vi "Pockels Cal-Wizard.vi"   [LabVIEW 2013]
uses:
  Configuration code/Calibration/AOL Z/Typedefs/Cal points.ctl
  User Interface/Windows/System config window/Typedefs/HW Setup tab control.ctl
  Configuration code/Calibration/Globals/gl_Calibration globals.vi
types:
  T1 = enum8{"Enabled", "Disabled", "Disabled and Grayed Out"}
  T2 = typedef "HW Setup tab control.ctl" = enum32{"Control system ", "Triggers", "DAQ FPGA", "HW Channels Setup", "XY stage", "Encoder", "System Setup", "Cameras", "AOL Properties", "Calibration Settings", "Reserved 1", "Reserved 2"}
  T3 = typedef "Cal points.ctl" = enum16{"5-points calibration (crude)", "11-points calibration", "21-points calibration", "41-points calibration"}
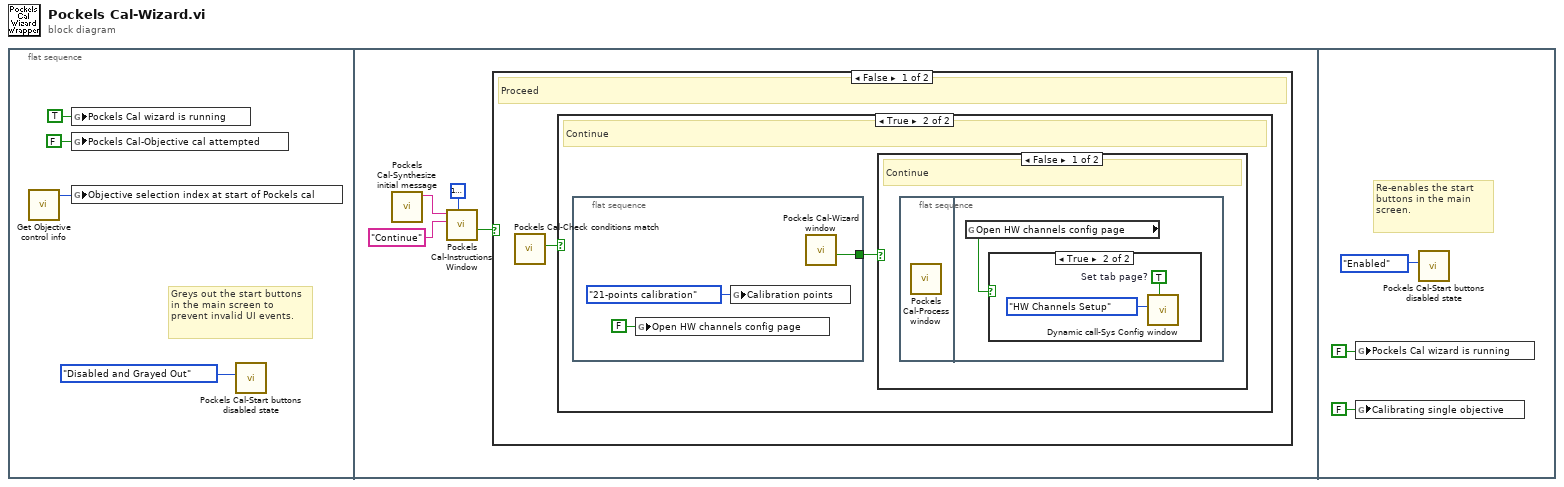
[diagram p0: block diagram]
diagram:
  n1 = flat-sequence {
    frame #0 {
      # "Greys out the start buttons in the main screen to prevent invalid UI events."
      n2 = call "Get Objective control info.vi"() -> ("Selection index"=w1:i32)  [unwired: 7 in, 4 out]
      n3 = global write "gl_Calibration globals.vi" "Pockels Cal wizard is running"(TRUE ("Motor Z Cal wizard is running")) -> ()
      n4 = global write "gl_Calibration globals.vi" "Pockels Cal-Objective cal attempted"(FALSE ("Pockels Cal-Objective cal attempted")) -> ()
      n5 = global write "gl_Calibration globals.vi" "Objective selection index at start of Pockels cal"(w1) -> ()
      n6 = call "Pockels Cal-Start buttons disabled state.vi"("Disabled"=T1."Disabled and Grayed Out") -> ()  [unwired: 10 in, 1 out]
    }
    frame #1 {
      n7 = call "Pockels Cal-Synthesize initial message.vi"() -> ("Message"=w6:string)  [unwired: 11 in]
      n8 = call "Pockels Cal-Instructions Window.vi"("Colour"=u32 16777225, "Caption-Right button (OK)"="Continue", "Message string"=w6) -> ("Cancelled (Left button pressed)"=w8:bool)  [unwired: 7 in, 1 out]
      n9 = case shown="False" w8 {
        frame False {
          # "Proceed"
          n10 = call "Pockels Cal-Check conditions match.vi"() -> ("Continue"=w9:bool)  [unwired: 11 in]
          n11 = case shown="True" w9 {
            frame False {
              # "Cancelled"
            }
            frame True {
              # "Continue"
              n12 = flat-sequence {
                tunnel: [w14] -> w10
                frame #0 {
                  n13 = global write "gl_Calibration globals.vi" "Open HW channels config page"(FALSE ("Open HW channels config page")) -> ()
                  n14 = global write "gl_Calibration globals.vi" "Calibration points"(Cal_points."21-points calibration" ("Calibration points")) -> ()
                  n15 = call "Pockels Cal-Wizard window.vi"() -> ("Cancelled"=w14:bool)  [unwired: 10 in, 1 out]
                }
              }
              n16 = case shown="False" w10 {
                frame False {
                  # "Continue"
                  n17 = flat-sequence {
                    frame #0 {
                      n18 = call "Pockels Cal-Process window.vi"() -> ()  [unwired: 10 in, 2 out]
                    }
                    frame #1 {
                      n19 = global read "gl_Calibration globals.vi" "Open HW channels config page"() -> (w11:bool)
                      n20 = case shown="True" w11 {
                        frame False {
                        }
                        frame True {
                          w12 = TRUE  # Set tab page?
                          n21 = call "Dynamic call-Sys Config window.vi"("Set tab page? (F)"=w12, "System Config Tab Control"=HW_Setup_tab_control."HW Channels Setup") -> ()  [unwired: 9 in, 1 out]
                        }
                      }
                    }
                  }
                }
                frame True {
                  # "Cancelled"
                }
              }
            }
          }
        }
        frame True {
          # "Cancelled"
        }
      }
    }
    frame #2 {
      # "Re-enables the start buttons in the main screen."
      n22 = global write "gl_Calibration globals.vi" "Pockels Cal wizard is running"(FALSE ("Motor Z Cal wizard is running")) -> ()
      n23 = global write "gl_Calibration globals.vi" "Calibrating single objective"(FALSE ("Calibrating single objective")) -> ()
      n24 = call "Pockels Cal-Start buttons disabled state.vi"("Disabled"=T1."Enabled") -> ()  [unwired: 10 in, 1 out]
    }
  }
